vi "Write Left Joystick Axis.vi"(8 "error in (no error)":errorcluster, 10 "Joystick Axis":T1 {"Y" scale=-1.0..1.0; "X" scale=-1.0..1.0}, 11 "XboxController-V in":refnum<class "XboxController-V.lvclass">) -> (0 "error out":errorcluster, 3 "XboxController-V out":refnum<class "XboxController-V.lvclass">)   [LabVIEW 2013, in "XboxController-V.lvclass"]
uses:
  XboxController-V.lvclass
  Logical Systems/XBoxController/JoystickAxis.ctl
  XboxController-V.lvclass/XboxController-V.ctl
  Logical Systems/XBoxController/XBoxController.lvclass
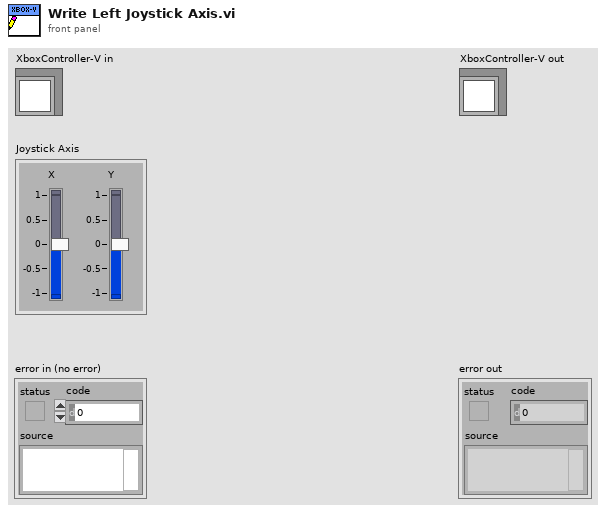
[diagram p1: front panel]
types:
  T1 = typedef "XBoxController.lvclass/JoystickAxis.ctl" = cluster{"X":dbl, "Y":dbl}
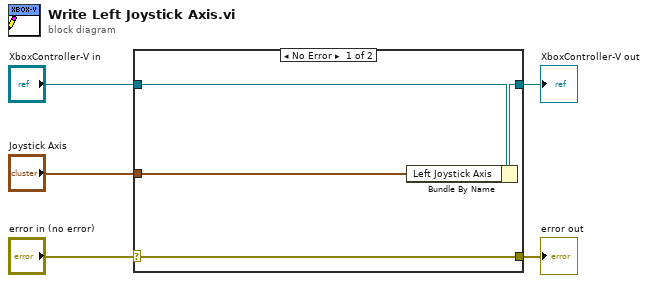
[diagram p0: block diagram]
diagram:
  n1 = case shown="No Error" "error in (no error)" {
    selector: "error in (no error)" -> [w9 w10]
    tunnel: [w9 w10] -> w4
    tunnel: [w7 w11] -> w2
    tunnel: "XboxController-V in" -> [w8 w11]
    tunnel: "Joystick Axis" -> [w6 _]
    frame No Error {
      n2 = Bundle By Name(cluster=w8, "Left Joystick Axis"=w6) -> (w7:refnum<class "XboxController-V.lvclass">)
    }
    frame Error {
    }
  }
  "error out" <- w4
  "XboxController-V out" <- w2
